vi "Graph Ref AE.vi"(7 "Action":enum16{"READ", "WRITE"}(ring), 10 "Graph Ref In":refnum<vi>[](array[refnum])) -> (2 "Graph Ref Out":refnum<vi>[](array[refnum]))   [LabVIEW 2015]
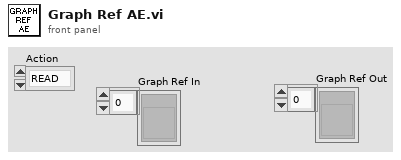
[diagram p1: front panel]
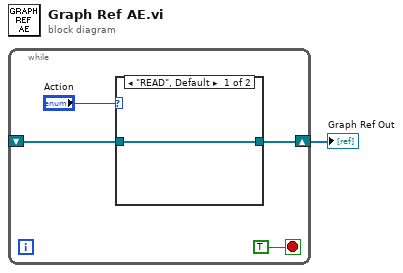
[diagram p0: block diagram]
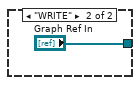
[diagram p2: hidden frame]
diagram:
  n1 = while {
    shift-right: [w4] -> w1
    shift-left: _ -> [w3]
    stop <- TRUE stop-if-true
    n2 = case shown="\"READ\", Default" "Action" {
      tunnel: [w6 "Graph Ref In"] -> w4
      tunnel: w3 -> [w6 _]
      frame "READ", Default {
      }
      frame "WRITE" {
      }
    }
  }
  "Graph Ref Out" <- w1
